vi "MPU.vi"   [LabVIEW 2018]
uses:
  <vilib>/rvi/Emulation/niFpgaGetClockAttributes.vi
  <vilib>/rvi/Emulation/niFpgaSctlEmulationGetInTimedLoop.vi
  <vilib>/rvi/Emulation/niFpgaEmulationReportErrorSimple.vi
  <vilib>/rvi/interface/RandomDataEmulation/niFpgaRandomDataHandleErrors.vi
  <vilib>/rvi/Emulation/niFpgaEmulationIsFPGAContextNoSignature.vi
  <vilib>/rvi/errors/niFpgaSetErrorForExecOnDevCompSimple.vi
  <vilib>/rvi/eio/common/nirviEmuReportErrorAndStop.vi
  <vilib>/rvi/DataTransferAndStorage/Container/Common/niFpgaContainerGetUniqueNameForEmu.vi
  <vilib>/rvi/FIFO/Fifo_Resource/nirvififoEmulationSetSize.vi
  <vilib>/rvi/FIFO/Fifo_Resource/nirviFifoEmulationQueueMgr.vi
  <instcachedir>/0/nirviFifoEmulationQueueMgr_E5CAEC123FF24DC58D834DCA3CDAA9B5.lvgen/nirviFifoEmulationQueueMgr_E5CAEC123FF24DC58D834DCA3CDAA9B5_001.vi
  <vilib>/rvi/FIFO/Fifo_Resource/nirvififoEmulationDetermineInputValidOut.vi
  <vilib>/rvi/FIFO/Fifo_Resource/nirvififoEmulationCreateLock.vi
  <vilib>/rvi/Emulation/niFpgaProcessEmulError.vi
  <vilib>/rvi/FIFO/Fifo_Resource/nirvififoEmulationObtainLock.vi
  <vilib>/rvi/FIFO/Fifo_Resource/nirvififoEmulationReleaseLock.vi
  <vilib>/rvi/occurrence/nirviWaitOnOccurrenceBase.vi
  <vilib>/rvi/errors/nirviReportUnexpectedCaseInternalError.vi
  <vilib>/rvi/errors/nirviReportUnexpectedCaseInternalError (U32).vi
  <vilib>/rvi/DataTransferAndStorage/Container/Common/niFpgaContainerExecOnDevCompGetState.vi
  <vilib>/Utility/error.llb/Clear Errors.vi
  <vilib>/rvi/Emulation/niFpgaCriticalErrorInLSC.vi
  <vilib>/rvi/DataTransferAndStorage/Container/XNode/niFpgaContainer.xnode
  <vilib>/rvi/interface/RandomDataEmulation/nirviRandomDataFpgaReadWriteTemplate.vi
  <vilib>/rvi/FIFO/Fifo_Resource/nirvififoEmulationWrite.vi
  <vilib>/rvi/FIFO/Fifo_Resource/niFpgaFifoEmulationRefIn.vi
  Modbus_Processing_Unit/src/MPU.lvclass
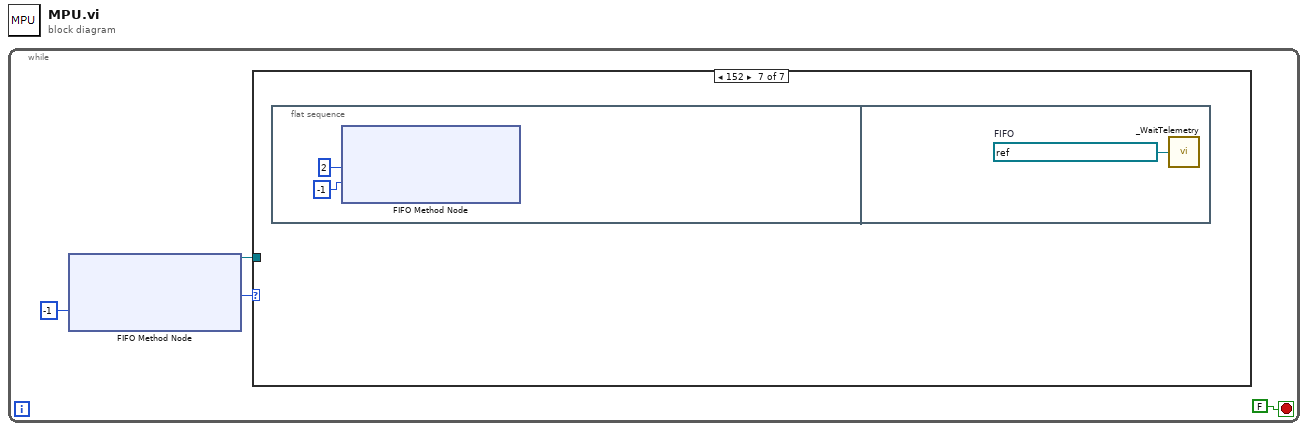
[diagram p0: block diagram]
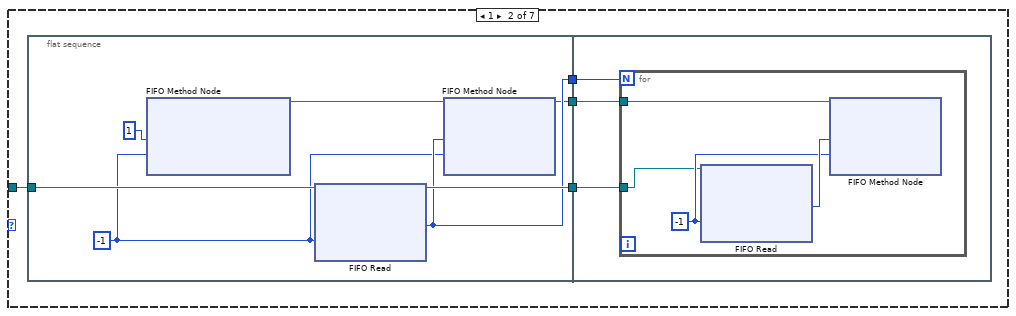
[diagram p3: hidden frame]
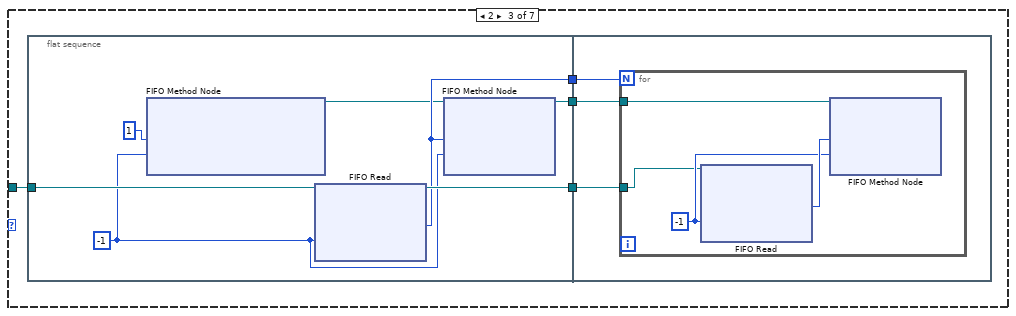
[diagram p4: hidden frame]
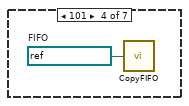
[diagram p5: hidden frame]
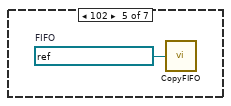
[diagram p6: hidden frame]
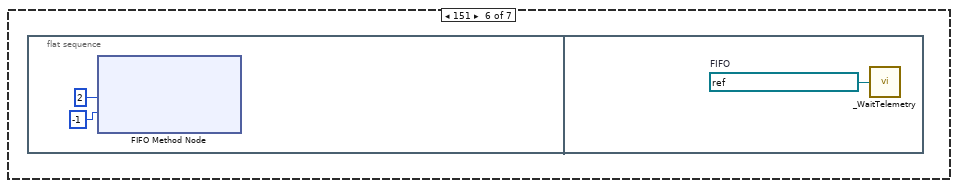
[diagram p7: hidden frame]
diagram:
  n1 = while {
    stop <- FALSE stop-if-true
    n2 = xnode ("FIFO Method Node")("Timeout"=-1) -> ("Element"=w4:u8, "FIFO Out"=w2:refnum<k21>)  [unwired: 1 in, 1 out]
    n3 = case shown="152" w4 {
      tunnel: w2 -> [_ w8 w26 _ _ _ _]
      frame 0, Default {
      }
      frame 1 {
        n4 = flat-sequence {
          tunnel: w8 -> [w15]
          tunnel: [w14] -> w7
          tunnel: [w13] -> w6
          tunnel: [w11] -> w5
          tunnel: w7 -> [w18]
          tunnel: w6 -> [w17]
          tunnel: w5 -> [w16]
          frame #0 {
            w9 = -1 ("Timeout")
            n5 = xnode ("FIFO Method Node")("Element"=u8 1, "Timeout"=w9) -> ("FIFO Out"=w12:refnum<k21>)  [unwired: 1 in, 1 out]
            n6 = xnode ("FIFO Read")("Timeout"=w9, "FIFO In"=w15) -> ("Element"=w13:u8, "FIFO Out"=w14:refnum<k21>)  [unwired: 1 out]
            n7 = xnode ("FIFO Method Node")("Element"=w13, "Timeout"=w9, "FIFO In"=w12) -> ("FIFO Out"=w11:refnum<k21>)  [unwired: 1 out]
          }
          frame #1 {
            n8 = for {
              N: w17 -> [_]
              tunnel: w18 -> [w20]
              tunnel: w16 -> [w19]
              w21 = -1 ("Timeout")
              n9 = xnode ("FIFO Read")("Timeout"=w21, "FIFO In"=w20) -> ("Element"=w22:u8)  [unwired: 2 out]
              n10 = xnode ("FIFO Method Node")("Element"=w22, "Timeout"=w21, "FIFO In"=w19) -> ()  [unwired: 2 out]
            }
          }
        }
      }
      frame 2 {
        n11 = flat-sequence {
          tunnel: w26 -> [w33]
          tunnel: [w32] -> w25
          tunnel: [w31] -> w24
          tunnel: [w29] -> w23
          tunnel: w25 -> [w36]
          tunnel: w24 -> [w35]
          tunnel: w23 -> [w34]
          frame #0 {
            w27 = -1 ("Timeout")
            n12 = xnode ("FIFO Method Node")("Element"=u8 1, "Timeout"=w27) -> ("FIFO Out"=w30:refnum<k21>)  [unwired: 1 in, 1 out]
            n13 = xnode ("FIFO Read")("Timeout"=w27, "FIFO In"=w33) -> ("Element"=w31:u8, "FIFO Out"=w32:refnum<k21>)  [unwired: 1 out]
            n14 = xnode ("FIFO Method Node")("Element"=w31, "Timeout"=w27, "FIFO In"=w30) -> ("FIFO Out"=w29:refnum<k21>)  [unwired: 1 out]
          }
          frame #1 {
            n15 = for {
              N: w35 -> [_]
              tunnel: w36 -> [w38]
              tunnel: w34 -> [w37]
              w39 = -1 ("Timeout")
              n16 = xnode ("FIFO Read")("Timeout"=w39, "FIFO In"=w38) -> ("Element"=w40:u8)  [unwired: 2 out]
              n17 = xnode ("FIFO Method Node")("Element"=w40, "Timeout"=w39, "FIFO In"=w37) -> ()  [unwired: 2 out]
            }
          }
        }
      }
      frame 101 {
        w41 = refnum<k21> "VFDDebug"  # FIFO
        n18 = call "CopyFIFO.vi"("Input"=w41) -> ()
      }
      frame 102 {
        w42 = refnum<k21> "FlowMeterDebug"  # FIFO
        n19 = call "CopyFIFO.vi"("Input"=w42) -> ()
      }
      frame 151 {
        n20 = flat-sequence {
          frame #0 {
            n21 = xnode ("FIFO Method Node")("Element"=2 ("Timeout"), "Timeout"=-1) -> ()  [unwired: 1 in, 2 out]
          }
          frame #1 {
            w45 = refnum<k21> "VFDTelemetryFIFO"  # FIFO
            n22 = call "_WaitTelemetry.vi"("FIFO"=w45) -> ()
          }
        }
      }
      frame 152 {
        n23 = flat-sequence {
          frame #0 {
            n24 = xnode ("FIFO Method Node")("Element"=2 ("Timeout"), "Timeout"=-1) -> ()  [unwired: 1 in, 2 out]
          }
          frame #1 {
            w48 = refnum<k21> "FlowMeterTelemetryFIFO"  # FIFO
            n25 = call "_WaitTelemetry.vi"("FIFO"=w48) -> ()
          }
        }
      }
    }
  }
